vi "Read Physical.vi"(8 "error in (no error)":errorcluster, 11 "HK Item in":refnum<class "HK Item.lvclass">) -> (0 "error out":errorcluster, 2 "Physical":T1, 3 "HK Item out":refnum<class "HK Item.lvclass">)   [LabVIEW 2019, in "HK Item.lvclass"]
uses:
  HK Item.lvclass
  HK Channel Settings Physical.ctl
  HK Item.lvclass/HK Item.ctl
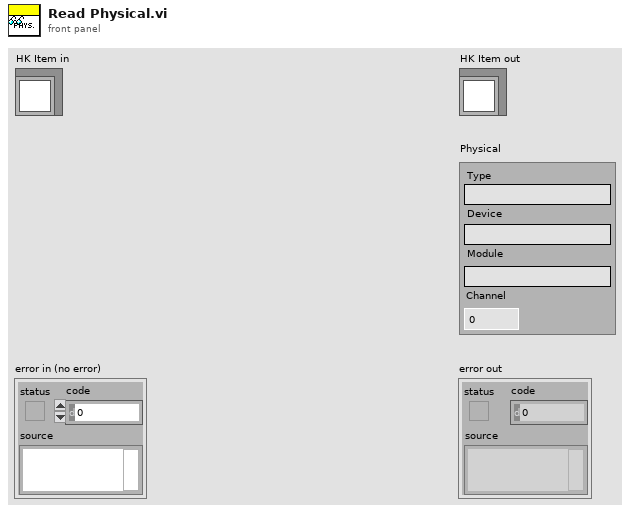
[diagram p1: front panel]
types:
  T1 = typedef "HK Item.lvclass/HK Channel Settings Physical.ctl" = cluster{"Type":string, "Device":string, "Module":string, "Channel":i32}
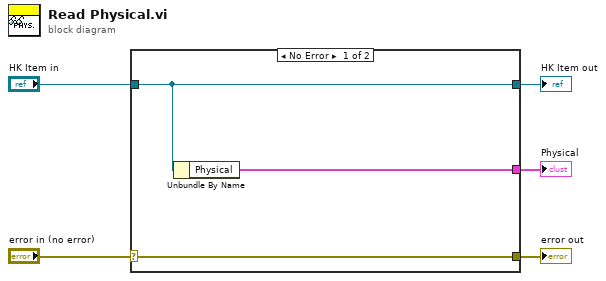
[diagram p0: block diagram]
diagram:
  n1 = case shown="No Error" "error in (no error)" {
    selector: "error in (no error)" -> [w8 w9]
    tunnel: [w8 w9] -> w4
    tunnel: [w7 w10] -> w2
    tunnel: "HK Item in" -> [w7 w10]
    tunnel: [w6 _] -> w1
    frame No Error {
      n2 = Unbundle By Name(w7) -> ("Physical"=w6:T1)
    }
    frame Error {
    }
  }
  "error out" <- w4
  "HK Item out" <- w2
  "Physical" <- w1
